vi "Read from TSM and Write to File Globals.vi"(0 "TSM context":T1, 5 "Sequence Ref In":refnum<k7>) -> (15 "error out":errorcluster)   [LabVIEW 2019]
uses:
  <vilib>/NI_TestStand_SemiconductorModule/NI_TestStand_Semiconductor_Module.lvlibp/PinMap/General/SemiconductorModuleContext.ctl
  <vilib>/NI_TestStand_SemiconductorModule/NI_TestStand_Semiconductor_Module.lvlibp
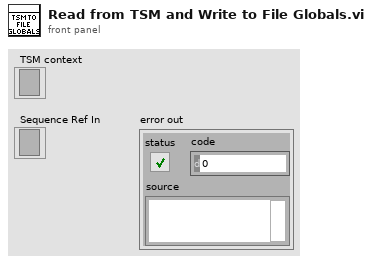
[diagram p1: front panel]
types:
  T1 = typedef "NI_TestStand_Semiconductor_Module.lvlibp/SemiconductorModuleContext.ctl" = refnum<k7>
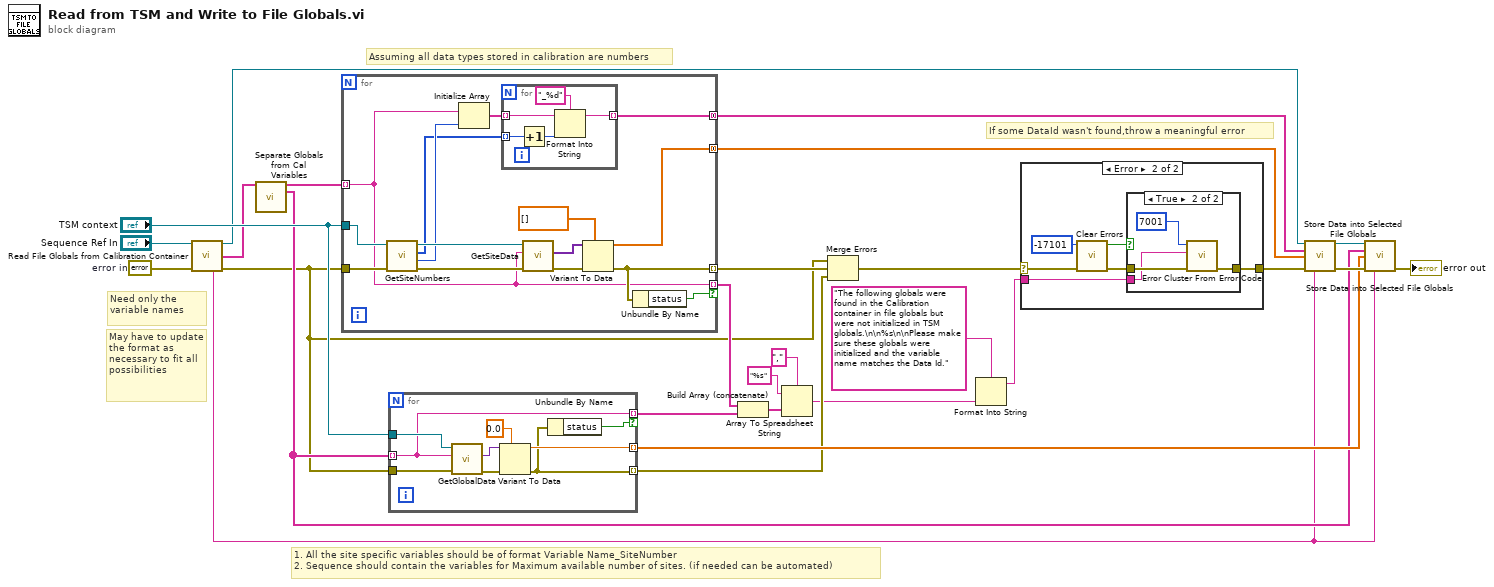
[diagram p0: block diagram]
diagram:
  w27 = errorcluster {"status"=FALSE, "code"=0, "source"=""}  # error in
  # "If some DataId wasn't found,throw a meaningful error"
  # "Assuming all data types stored in calibration are numbers"
  # "May have to update the format as necessary to fit all possibilities"
  # "1. All the site specific variables should be of format Variable Name_SiteNumber\n2. Sequence should contain the variables for Maximum available number of sites. (if needed can be automated)"
  # "Need only the variable names"
  n1 = call "Read File Globals from Calibration Container.vi"("Sequence Ref In"="Sequence Ref In", "error in"=w27) -> ("Sequence Ref Out"=w23:refnum<k7>, "Calibration Variables"=w17:string[], "lookupString"=w1:string, "error out"=w4:errorcluster)  [unwired: 8 in, 2 out]
  n2 = call "Separate Globals from Cal Variables.vi"("Calibration Variables"=w17) -> ("Site Globals"=w16:string[], "Globals"=w15:string[])  [unwired: 13 in]
  n3 = for {
    tunnel: "TSM context" -> [w36]
    tunnel: w16 -> [w29] mode=indexing
    tunnel: [w38] -> w21 mode=concatenating
    tunnel: [w31] -> w22 mode=concatenating
    tunnel: w4 -> [w42]
    tunnel: [w30] -> w24 mode=indexing
    tunnel: [w29] -> w10 mode=indexing if=w28
    n4 = call <vilib>:"GetSiteNumbers.vi"("error in (no error)"=w42, "Semiconductor Module Context"=w36) -> ("error out"=w37:errorcluster, "Number Of Sites"=w34:i32, "Site Numbers"=w32:i32[], "Semiconductor Module Context Out"=w35:T1)  [unwired: 6 in]
    n5 = Initialize Array(w29, w34) -> (w33:string[])
    n6 = for {
      tunnel: w33 -> [w47] mode=indexing
      tunnel: w32 -> [w46] mode=indexing
      tunnel: [w44] -> w31 mode=indexing
      n7 = Increment(x=w46) -> (x+1=w43:i32)
      n8 = Format Into String(format string="_%d", initial string=w47, w43) -> (resulting string=w44:string)  [unwired: 1 in, 1 out]
    }
    n9 = call <vilib>:"GetSiteData.vi"("error in (no error)"=w37, "Data Id"=w29, "Semiconductor Module Context"=w35) -> ("error out"=w41:errorcluster, "Site Data"=w40:variant[])  [unwired: 6 in, 1 out]
    n10 = Variant To Data(error in=w41, type=dbl[] [], Variant=w40) -> (data=w38:dbl[], error out=w30:errorcluster)
    n11 = Unbundle By Name(w30) -> ("status"=w28:bool)
  }
  n12 = for {
    tunnel: "TSM context" -> [w55]
    tunnel: w15 -> [w49] mode=indexing
    tunnel: [w51] -> w18 mode=indexing
    tunnel: w4 -> [w56]
    tunnel: [w50] -> w13 mode=indexing
    tunnel: [w49] -> w9 mode=indexing if=w48
    n13 = call <vilib>:"GetGlobalData.vi"("error in (no error)"=w56, "Data Id"=w49, "Semiconductor Module Context"=w55) -> ("error out"=w54:errorcluster, "Data"=w53:variant)  [unwired: 6 in, 1 out]
    n14 = Variant To Data(error in=w54, type=0.0, Variant=w53) -> (data=w51:dbl, error out=w50:errorcluster)
    n15 = Unbundle By Name(w50) -> ("status"=w48:bool)
  }
  n16 = Build Array (concatenate)(w10, w9) -> (w8:string[])
  n17 = Array To Spreadsheet String(delimiter (Tab)=",", array=w8, 3:"%s" ("format string")) -> (spreadsheet string=w5:string)
  n18 = Merge Errors(w4, w24, w13) -> (w12:errorcluster)
  n19 = Format Into String(format string="The following globals were found in the Calibration container in file globals but were not initialized in TSM globals.\n\n%s\n\nPlease make sure these globals were initialized and the variable name matches the Data Id." ("string"), w5) -> (resulting string=w2:string)  [unwired: 2 in, 1 out]
  n20 = case shown="Error" w12 {
    selector: w12 -> [w57 w63]
    tunnel: [w57 w62] -> w11
    tunnel: w2 -> [_ w58]
    frame No Error {
    }
    frame Error {
      n21 = call <vilib>:"Clear Errors.vi"("error in (no error)"=w63, "specific error code to clear (0: all)"=-17101) -> ("error out"=w61:errorcluster, "specific error cleared?"=w60:bool)  [unwired: 4 in]
      n22 = case shown="True" w60 {
        tunnel: w61 -> [w64 w68]
        tunnel: [w64 w67] -> w62
        tunnel: w58 -> [_ w65]
        frame False {
        }
        frame True {
          n23 = call <vilib>:"Error Cluster From Error Code.vi"("error in (no error)"=w68, "error message (\"\")"=w65, "error code (0)"=7001) -> ("error out"=w67:errorcluster)  [unwired: 6 in]
        }
      }
    }
  }
  n24 = call "Store Data into Selected File Globals.vi"("Sequence Ref In"=w23, "Variable Names"=w22, "Values to Set"=w21, "error in"=w11, "lookupString"=w1) -> ("Sequence Ref Out"=w19:refnum<k7>, "error out"=w20:errorcluster)  [unwired: 9 in]
  n25 = call "Store Data into Selected File Globals.vi"("Sequence Ref In"=w19, "Variable Names"=w15, "Values to Set"=w18, "error in"=w20, "lookupString"=w1) -> ("error out"=→"error out":errorcluster)  [unwired: 9 in, 1 out]
